vi "Copy_UI_Data.vi"(8 "error in (no error)":errorcluster, 10 "IB_Source in":refnum<class "IB_Source.lvclass">, 11 "IB_TreeSrcItem.lvclass":refnum<class "IB_Tree_Item_Source_File.lvclass">) -> (0 "error out":errorcluster, 3 "IB_TreeSrcItem out":refnum<class "IB_Tree_Item_Source_File.lvclass">)   [LabVIEW 2020, in "IB_Tree_Item_Source_File.lvclass"]
uses:
  <vilib>/AppBuilder/IB_Classes/Tree_Item_Source_File/IB_Tree_Item_Source_File.lvclass
  <vilib>/AppBuilder/IB_Classes/Tree_Item_Source_File/IB_Tree_Item_Source_File.lvclass/IB_Tree_Item_Source_File.ctl
  <vilib>/AppBuilder/IB_Classes/Source/IB_Source.lvclass
  <vilib>/AppBuilder/IB_Classes/Tree_Item/IB_Tree_Item.lvclass
  e:/builds/penguin/labview/branches/2020/dev/dist/vi.lib/AppBuilder/IB_Classes/Tree_Item_Source/IB_Tree_Item_Source.lvclass
  e:/builds/penguin/labview/branches/2020/dev/dist/vi.lib/AppBuilder/IB_Classes/Tree_Item/IB_Tree_Item.lvclass
  e:/builds/penguin/labview/branches/2020/dev/dist/vi.lib/AppBuilder/IB_Classes/Tree_Item_Source_File/IB_Tree_Item_Source_File.lvclass
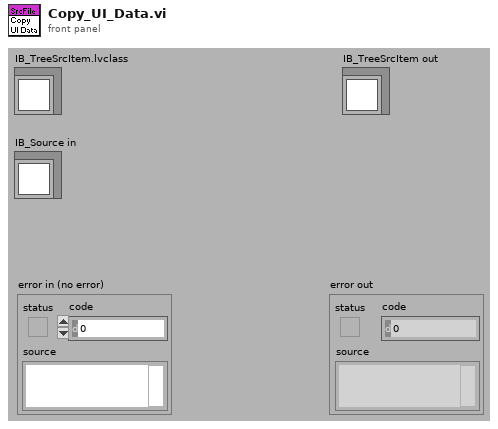
[diagram p1: front panel]
types:
  T1 = typedef "IB_Source.ctl" = cluster{"name":string, "sourceTag":string, "destTag":string, "path":path, "eng_installPath":string, "UI_inBuild?":bool, "str ref?":bool}
  T2 = typedef "IB_Tree_Item.ctl" = cluster{"symbol index":i32, "child tag":string, "parentTag":string, "left cell name":string}
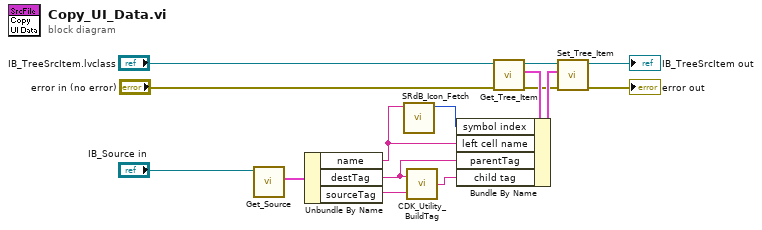
[diagram p0: block diagram]
diagram:
  n1 = call <vilib>:"Get_Source.vi"("IB_Source in"="IB_Source in") -> ("data"=w14:T1)  [unwired: 8 in, 2 out]
  n2 = Unbundle By Name(w14) -> ("name"=w4:string, "destTag"=w12:string, "sourceTag"=w15:string)
  n3 = call <resource>:"SRdB_Icon_Fetch.vi"("filename"=w4) -> ("symbol index"=w3:i32)  [unwired: 8 in, 2 out]
  n4 = call <resource>:"CDK_Utility_BuildTag.vi"("name or relative path"=w15, "BasePath"=w12) -> ("appended path"=w13:string)
  n5 = call <vilib>:"Get_Tree_Item.vi"("error in (no error)"="error in (no error)", "IB_TreeItem in"="IB_TreeSrcItem.lvclass") -> ("error out"=w7:errorcluster, "data"=w10:T2, "IB_TreeItem out"=w11:refnum<class "IB_Tree_Item_Source_File.lvclass">)  [unwired: 7 in]
  n6 = Bundle By Name(cluster=w10, "symbol index"=w3, "left cell name"=w4, "parentTag"=w12, "child tag"=w13) -> (w9:T2)
  n7 = call <vilib>:"Set_Tree_Item.vi"("error in (no error)"=w7, "data"=w9, "IB_TreeItem in"=w11) -> ("error out"=→"error out":errorcluster, "IB_TreeItem out"=→"IB_TreeSrcItem out":refnum<class "IB_Tree_Item_Source_File.lvclass">)  [unwired: 7 in]
